vi "Refresh Configuration File.vi"(8 "error in":errorcluster, 9 "Path":path, 10 "Name":string, 11 "Database section Ref":T1 format="%.0x") -> (0 "error out":errorcluster, 3 "Database Ref out":T1 format="%.0x")   [LabVIEW 2020, in "Ballard ARINC 429 Scripting.lvlib"]
uses:
  <vilib>/NI VeriStand/Custom Device API/Custom Device Item Ref.ctl
  Constants.vi
  <vilib>/NI VeriStand/Custom Device API/Set Item Property (Path).vi
  Ballard ARINC 429 Scripting.lvlib
  <vilib>/NI VeriStand/Custom Device API/Custom Device API.lvlib
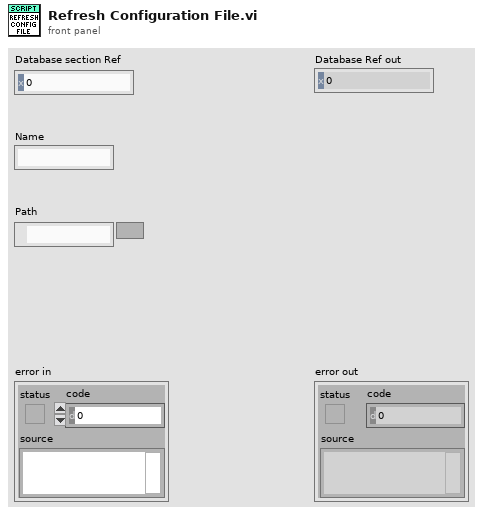
[diagram p1: front panel]
types:
  T1 = typedef "Custom Device API.lvlib/Custom Device Item Ref.ctl" = u64
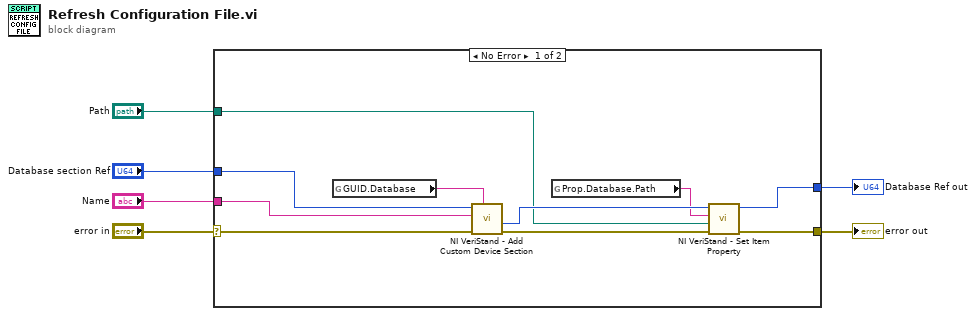
[diagram p0: block diagram]
diagram:
  n1 = case shown="No Error" "error in" {
    selector: "error in" -> [w10 w17]
    tunnel: "Name" -> [w14 _]
    tunnel: "Database section Ref" -> [w13 _]
    tunnel: [w12 w17] -> w4
    tunnel: "Path" -> [w11 _]
    tunnel: [w9 _] -> w1
    frame No Error {
      n2 = global read "Constants.vi" "GUID.Database"() -> (w8:string)
      n3 = call <vilib>:"NI VeriStand - Add Custom Device Section.vi"("GUID (Default Section)"=w8, "error in (no error)"=w10, "Section Name"=w14, "Parent Ref in"=w13) -> ("error out"=w15:errorcluster, "Section Ptr"=w16:T1)  [unwired: 4 in, 2 out]
      n4 = global read "Constants.vi" "Prop.Database.Path"() -> (w7:string)
      n5 = call-poly <vilib>:"NI VeriStand - Set Item Property.vi"("error in (no error)"=w15, "Value"=w11, "Property Name"=w7, "Item Ref in"=w16) -> ("error out"=w12:errorcluster, "Item Ref out"=w9:T1)  [unwired: 5 in, 1 out]
    }
    frame Error {
    }
  }
  "error out" <- w4
  "Database Ref out" <- w1
